vi "SetOutput.vi"(8 "error in (no error)":errorcluster, 9 "Boolean":bool=TRUE, 10 "Index":i32, 11 "IOCard in":refnum<class "IOCard.lvclass">) -> (0 "error out":errorcluster, 1 "life+1":bool, 3 "IOCard out":refnum<class "IOCard.lvclass">)   [LabVIEW 2019, in "IOCard.lvclass"]
uses:
  IOCard.lvclass
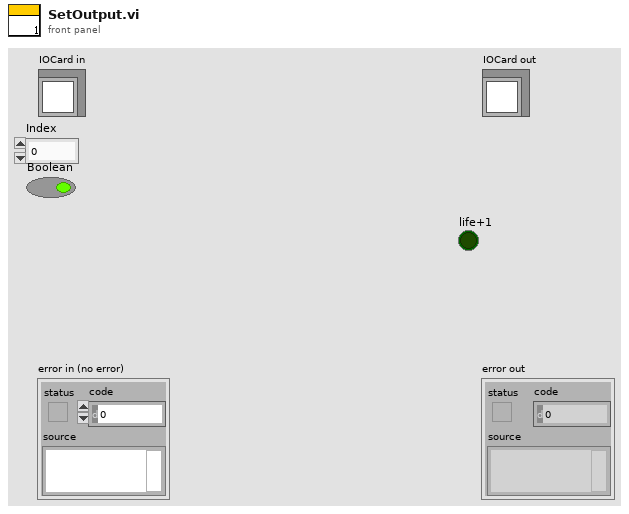
[diagram p1: front panel]
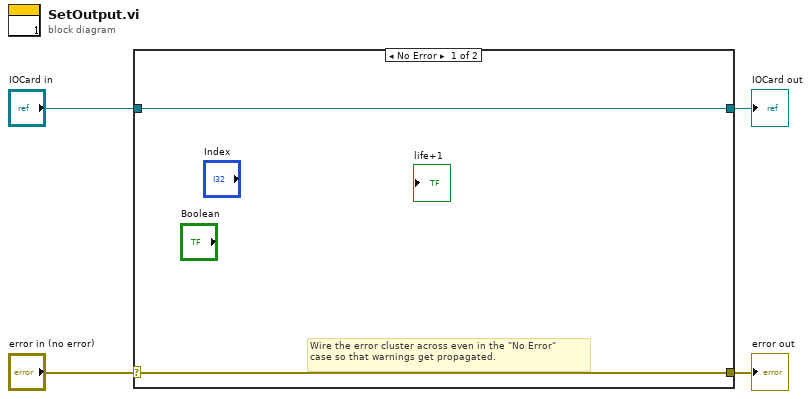
[diagram p0: block diagram]
diagram:
  n1 = case shown="No Error" "error in (no error)" {
    selector: "error in (no error)" -> [w5 w8]
    tunnel: [w5 w8] -> w3
    tunnel: [w6 w7] -> w1
    tunnel: "IOCard in" -> [w6 w7]
    frame No Error {
      # "Wire the error cluster across even in the \"No Error\"\ncase so that warnings get propagated."
    }
    frame Error {
    }
  }
  "error out" <- w3
  "IOCard out" <- w1
